vi "Main.vi"() -> ()   [LabVIEW 2019]
uses:
  Typedefs/#enum_MasterState.ctl
  Typedefs/#cluster_GUIRefs.ctl
  <vilib>/ActorFramework/Message Enqueuer/Message Enqueuer.lvclass/Message Enqueuer.ctl
  ViewerManager/ViewerManager Messages/UpdateMeasurementDirectory Msg/UpdateMeasurementDirectory Msg.lvclass/UpdateMeasurementDirectory Msg.ctl
  SubVIs/Application Configuration VIs/#cluster_AppConfiguration.ctl
  <vilib>/ActorFramework/Message Enqueuer/Enqueue.vi
  <vilib>/ActorFramework/Stop Msg/Stop Msg.lvclass
  C:/Program Files (x86)/National Instruments/LabVIEW 2019/vi.lib/ActorFramework/Message/Message.lvclass
  ViewerManager/ViewerManager Messages/UpdateMeasurementDirectory Msg/UpdateMeasurementDirectory Msg.lvclass
  ViewerManager/ViewerManager Messages/ShowViewer Msg/ShowViewer Msg.lvclass
  <vilib>/Utility/LVClass/Get LV Class Name.vi
  <resource>/AFDebug/Generate Trace for Message.vi
  <vilib>/ActorFramework/Message Priority Queue/Priority Enqueue.vi
  SubVIs/LowLevelError.vi
panel:
  in  "Results Viewer":bool
  in  "POX Data History":string[](array[string])
  in  "Save?":bool caption="Save Results?"
  in  "Measure":bool
  in  "Measurement Directory":path
  in  "Stop":bool
  out "O2 Saturation":dbl(graph)
  out "Heart beat":dbl(graph)
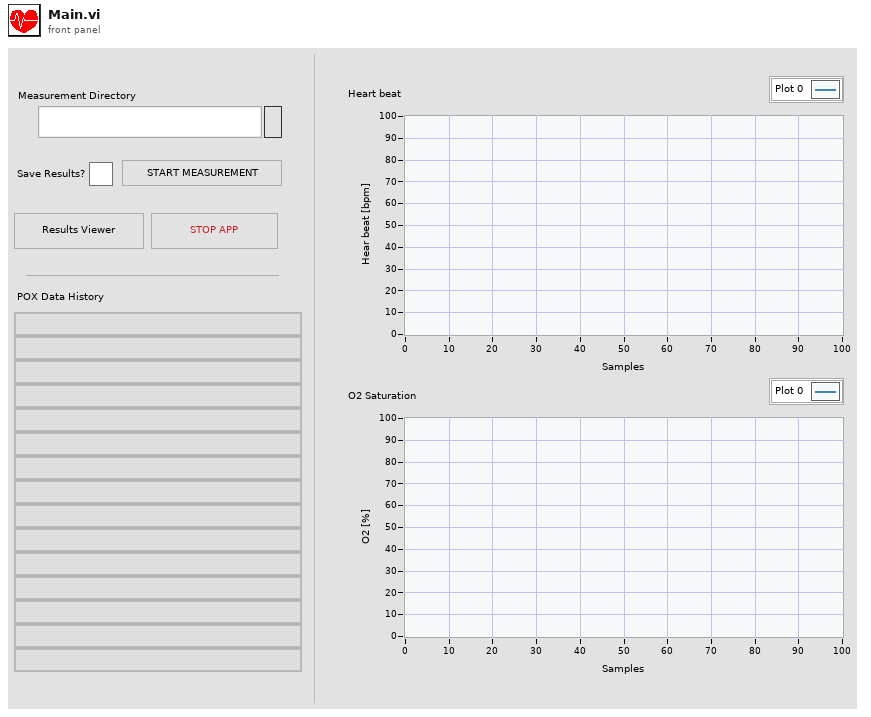
[diagram p1: front panel]
types:
  T1 = typedef "#enum_MasterState.ctl" = enum16{"Idle", "Init", "Close", "Error"}
  T2 = typedef "#cluster_ApplicationData.ctl" = cluster{"Acq Queue":refnum<queue>, "Saving Queue":refnum<queue>, "Viewer Manager Enqueuer":refnum<class "Message Enqueuer.lvclass">}
  T3 = typedef "#cluster_GUIRefs.ctl" = cluster{"Measure":refnum<vi>, "Save?":refnum<vi>, "Stop":refnum<vi>, "Measurement Dir":refnum<vi>, "Heart beat":refnum<vi>, "O2":refnum<vi>, "POX Data History":refnum<vi>}
  T4 = typedef "#cluster_AppConfiguration.ctl" = cluster{"Measurements Directory":path}
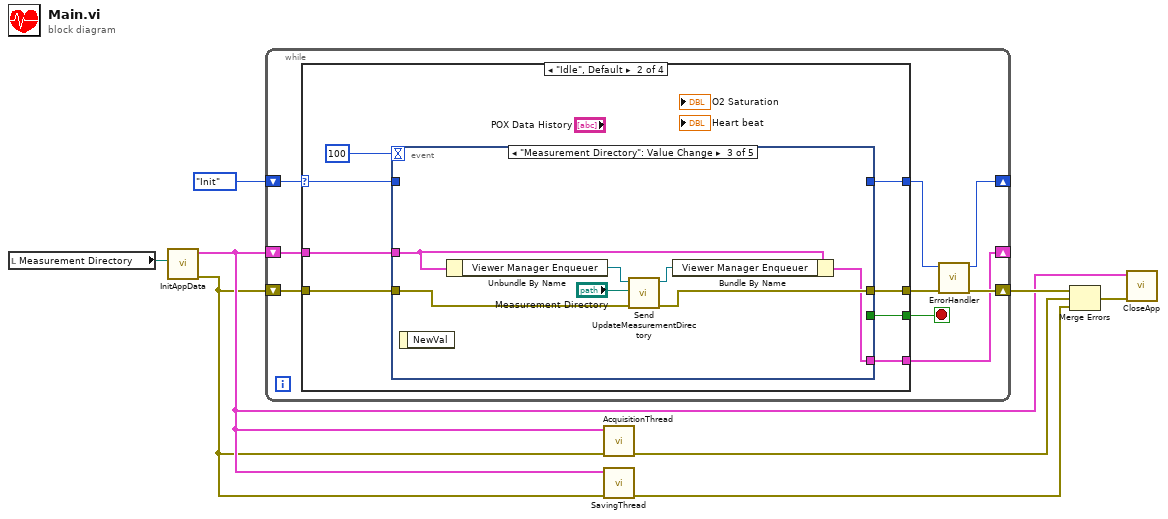
[diagram p0: block diagram]
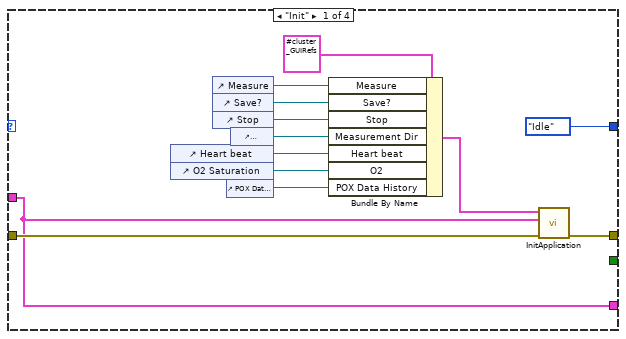
[diagram p2: hidden frame]
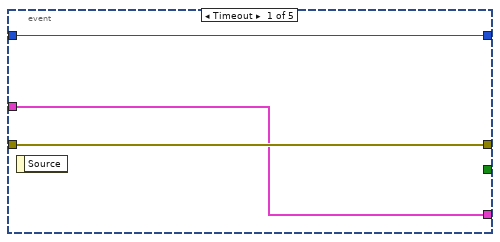
[diagram p3: hidden frame]
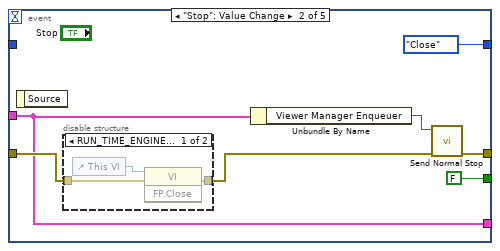
[diagram p4: hidden frame]
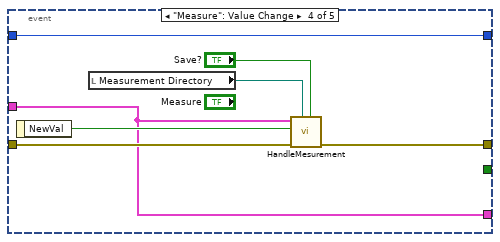
[diagram p6: hidden frame]
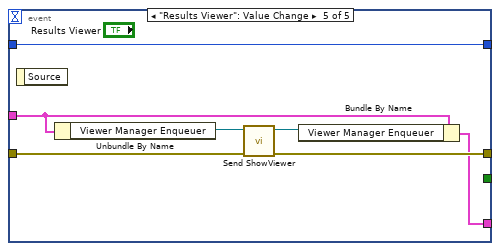
[diagram p7: hidden frame]
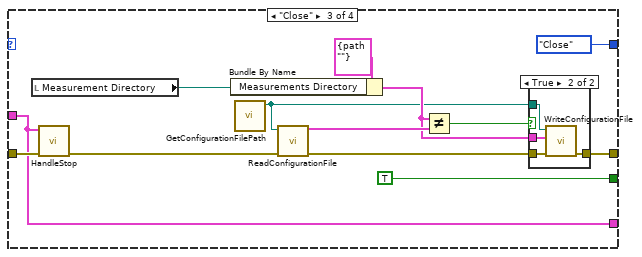
[diagram p8: hidden frame]
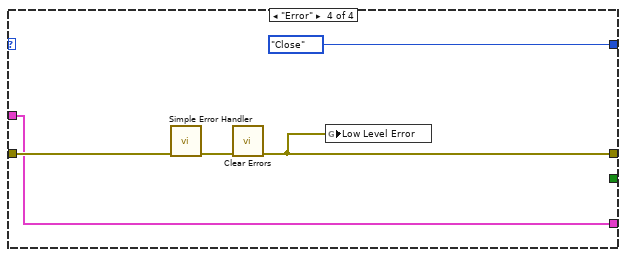
[diagram p10: hidden frame]
diagram:
  n1 = local read "Measurement Directory"() -> (w1:path)
  n2 = call "InitAppData.vi"("Measurement Directory"=w1) -> ("error out"=w2:errorcluster, "Application Data"=w3:T2)  [unwired: 9 in]
  n3 = while {
    shift-right: [w12] -> w8
    shift-left: w2 -> [w17]
    shift-right: [w10] -> _
    shift-left: #enum_MasterState."Init" ("Master State") -> [w14]
    shift-right: [w9] -> _
    shift-left: w3 -> [w16]
    stop <- w15 stop-if-true
    n4 = case shown="\"Idle\", Default" w14 {
      selector: w14 -> [_ w35 _ _]
      tunnel: w17 -> [w23 w38 w86 w95]
      tunnel: w16 -> [w18 w32 w74 w92]
      tunnel: [w21 w37 w80 w93] -> w13
      tunnel: [_ w36 TRUE _] -> w15
      tunnel: [#enum_MasterState."Idle" ("Master State") w34 #enum_MasterState."Close" ("Master State") #enum_MasterState."Close" ("Master State")] -> w11
      tunnel: [w18 w31 w74 w92] -> w9
      frame "Init" {
        n5 = control-ref of="Heart beat"() -> (w29:refnum<vi>)
        n6 = control-ref of="O2 Saturation"() -> (w30:refnum<vi>)
        n7 = control-ref of="Measure"() -> (w25:refnum<vi>)
        n8 = control-ref of="Save?"() -> (w26:refnum<vi>)
        n9 = control-ref of="Stop"() -> (w27:refnum<vi>)
        n10 = control-ref of="POX Data History"() -> (w19:refnum<vi>)
        n11 = control-ref of="Measurement Directory"() -> (w28:refnum<vi>)
        n12 = Bundle By Name(cluster=T3 {"Measure"=refnum, "Save?"=refnum, "Stop"=refnum, "Measurement Dir"=refnum, "Heart beat"=refnum, "O2"=refnum, "POX Data History"=refnum} ("GUI Refs"), "Measure"=w25, "Save?"=w26, "Stop"=w27, "Measurement Dir"=w28, "Heart beat"=w29, "O2"=w30, "POX Data History"=w19) -> (w22:T3)
        n13 = call "InitApplication.vi"("error in (no error)"=w23, "Application Data in"=w18, "GUI Refs"=w22) -> ("error out"=w21:errorcluster)  [unwired: 8 in]
      }
      frame "Idle", Default {
        n14 = event shown="[2] \"Measurement Directory\": Value Change" {
          selector: _ -> [_ _ _ _ _]
          dyn-events: _ -> [_ _ _ _ _]
          timeout: 100 -> [_ _ _ _ _]
          tunnel: w38 -> [w41 w48 w57 w66 w73]
          tunnel: w32 -> [w39 w43 w59 w61 w70]
          tunnel: [w41 w44 w56 w64 w71] -> w37
          tunnel: [_ FALSE _ _ _] -> w36
          tunnel: w35 -> [w40 _ _ w62 w72]
          tunnel: [w40 #enum_MasterState."Close" ("Master State") _ w62 w72] -> w34
          tunnel: [w39 w43 w54 w61 w68] -> w31
          event Timeout {
            n15 = event-data() -> ()  [unwired: 1 in, 1 out]
          }
          event "Stop": Value Change {
            n16 = event-data() -> ()  [unwired: 1 in, 1 out]
            n17 = disable-structure shown="RUN_TIME_ENGINE==True" {
              disable-tunnel: w48 -> [w51 w52]
              disable-tunnel: [w50 w52] -> w45
              frame condition #0 {
                n18 = control-ref of="This VI"() -> (w49:refnum<vi>)
                n19 = invoke class="VI" method="FP.Close"(reference=w49, error in=w51) -> (error out=w50:errorcluster)  [unwired: 1 in, 2 out]
              }
              frame condition #1 (active) {
              }
            }
            n20 = Unbundle By Name(w43) -> ("Viewer Manager Enqueuer"=w42:refnum<class "Message Enqueuer.lvclass">)
            n21 = call <vilib>:"Send Normal Stop.vi"("error in (no error)"=w45, "Message Enqueuer"=w42) -> ("error out"=w44:errorcluster)  [unwired: 9 in]
          }
          event "Measurement Directory": Value Change {
            n22 = event-data() -> ()  [unwired: 1 in, 1 out]
            n23 = Unbundle By Name(w59) -> ("Viewer Manager Enqueuer"=w58:refnum<class "Message Enqueuer.lvclass">)
            n24 = call "Send UpdateMeasurementDirectory.vi"("error in (no error)"=w57, "Measurement Directory"="Measurement Directory", "Message Enqueuer"=w58) -> ("error out"=w56:errorcluster, "Message Enqueuer out"=w53:refnum<class "Message Enqueuer.lvclass">)  [unwired: 7 in]
            n25 = Bundle By Name(cluster=w59, "Viewer Manager Enqueuer"=w53) -> (w54:T2)
          }
          event "Measure": Value Change {
            n26 = event-data() -> ("NewVal"=w65:bool)  [unwired: 1 in]
            n27 = local read "Measurement Directory"() -> (w60:path)
            n28 = call "HandleMesurement.vi"("Save?"="Save?", "Measurement Directory"=w60, "error in (no error)"=w66, "Measure?"=w65, "Application Data"=w61) -> ("error out"=w64:errorcluster)  [unwired: 6 in]
          }
          event "Results Viewer": Value Change {
            n29 = event-data() -> ()  [unwired: 1 in, 1 out]
            n30 = Unbundle By Name(w70) -> ("Viewer Manager Enqueuer"=w69:refnum<class "Message Enqueuer.lvclass">)
            n31 = call "Send ShowViewer.vi"("error in (no error)"=w73, "Message Enqueuer"=w69) -> ("error out"=w71:errorcluster, "Message Enqueuer out"=w67:refnum<class "Message Enqueuer.lvclass">)  [unwired: 8 in]
            n32 = Bundle By Name(cluster=w70, "Viewer Manager Enqueuer"=w67) -> (w68:T2)
          }
        }
      }
      frame "Close" {
        n33 = local read "Measurement Directory"() -> (w78:path)
        n34 = call "HandleStop.vi"("error in (no error)"=w86, "Application Data"=w74) -> ("error out"=w83:errorcluster)  [unwired: 9 in]
        n35 = Bundle By Name(cluster=T4 {"Measurements Directory"=path ""} ("App Configuration"), "Measurements Directory"=w78) -> (w76:T4)
        n36 = call "GetConfigurationFilePath.vi"() -> ("Configuration File Path"=w75:path)  [unwired: 11 in]
        n37 = call "ReadConfigurationFile.vi"("Error in"=w83, "Configuration File Path"=w75) -> ("Error out"=w82:errorcluster, "App Configuration"=w77:T4)  [unwired: 8 in]
        n38 = Not Equal?(x=w76, y=w77) -> (x != y?=w81:bool)
        n39 = case shown="True" w81 {
          tunnel: w82 -> [w87 w91]
          tunnel: [w87 w90] -> w80
          tunnel: w76 -> [_ w89]
          tunnel: w75 -> [_ w88]
          frame False {
          }
          frame True {
            n40 = call "WriteConfigurationFile.vi"("Error in"=w91, "App Configuration"=w89, "Configuration File Path"=w88) -> ("Error out"=w90:errorcluster)  [unwired: 8 in]
          }
        }
      }
      frame "Error" {
        n41 = call <vilib>:"Simple Error Handler.vi"("error in (no error)"=w95) -> ("error out"=w94:errorcluster)  [unwired: 4 in, 4 out]
        n42 = call <vilib>:"Clear Errors.vi"("error in (no error)"=w94) -> ("error out"=w93:errorcluster)  [unwired: 5 in, 1 out]
        n43 = global write "LowLevelError.vi" "Low Level Error"(w93) -> ()
      }
    }
    n44 = call "ErrorHandler.vi"("error in (no error)"=w13, "Master State in"=w11) -> ("error out"=w12:errorcluster, "Master State out"=w10:T1)  [unwired: 8 in]
  }
  n45 = call "AcquisitionThread.vi"("error in (no error)"=w2, "Application Data"=w3) -> ("error out"=w7:errorcluster)  [unwired: 9 in]
  n46 = call "SavingThread.vi"("error in (no error)"=w2, "Application Data"=w3) -> ("error out"=w5:errorcluster)  [unwired: 9 in]
  n47 = Merge Errors(w8, w7, w5) -> (w4:errorcluster)
  n48 = call "CloseApp.vi"("error in (no error)"=w4, "Application Data"=w3) -> ()  [unwired: 9 in, 1 out]
